vi "get_bias_spectroscopy_sweep_time.vi"() -> (0 "Sweep time (s)":sgl)   [LabVIEW 2021]
uses:
  <userlib>/Nanonis Prog Interface V5/Nanonis Prog Interface.lvlib
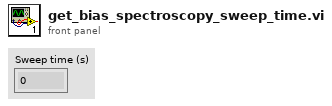
[diagram p1: front panel]
types:
  T1 = cluster{"Z averaging time (s)":sgl, "Z offset (m)":sgl, "Initial settling time (s)":sgl}
  T2 = cluster{"Max. slew rate (V/s)":sgl, "Settling time (s)":sgl, "Integration time (s)":sgl}
  T3 = cluster{"End settling time (s)":sgl, "Z control time (s)":sgl}
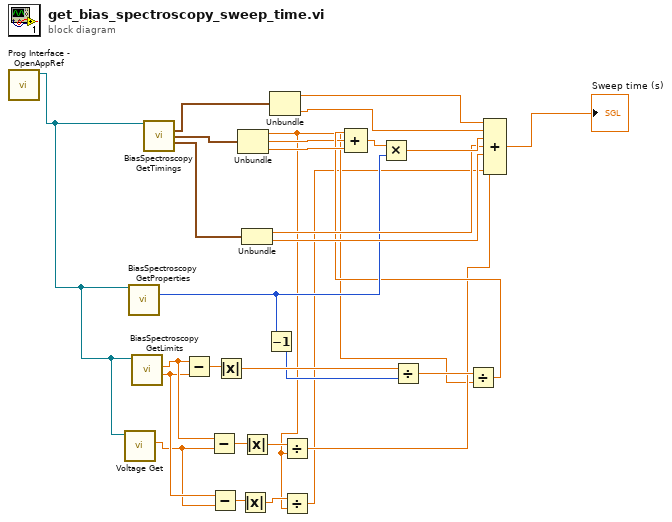
[diagram p0: block diagram]
diagram:
  n1 = call <userlib>:"Prog Interface - OpenAppRef.vi"() -> ("Application reference"=w12:refnum<vi>)  [unwired: 6 in, 1 out]
  n2 = call <userlib>:"Voltage Get.vi"("Application ref in"=w12) -> ("Bias (V)"=w5:sgl)  [unwired: 8 in, 2 out]
  n3 = call <userlib>:"BiasSpectroscopy GetProperties.vi"("Application ref in"=w12) -> ("Number of points"=w17:i32)  [unwired: 7 in, 7 out]
  n4 = call <userlib>:"BiasSpectroscopy GetLimits.vi"("Application ref in"=w12) -> ("End value (V)"=w6:sgl, "Start value (V)"=w11:sgl)  [unwired: 5 in, 2 out]
  n5 = call <userlib>:"BiasSpectroscopy GetTimings.vi"("Application ref in"=w12) -> ("Initialization"=w29:T1, "Sweep Timing"=w28:T2, "End of Sweep"=w27:T3)  [unwired: 10 in, 2 out]
  n6 = Subtract(x=w11, y=w6) -> (x-y=w19:sgl)
  n7 = Subtract(x=w11, y=w5) -> (x-y=w10:sgl)
  n8 = Subtract(x=w6, y=w5) -> (x-y=w4:sgl)
  n9 = Absolute Value(x=w19) -> (abs(x)=w18:sgl)
  n10 = Unbundle(w28) -> ("Max. slew rate (V/s)"=w2:sgl, "Settling time (s)"=w8:sgl, "Integration time (s)"=w26:sgl)
  n11 = Absolute Value(x=w4) -> (abs(x)=w3:sgl)
  n12 = Unbundle(w27) -> ("End settling time (s)"=w22:sgl, "Z control time (s)"=w21:sgl)
  n13 = Absolute Value(x=w10) -> (abs(x)=w9:sgl)
  n14 = Decrement(x=w17) -> (x-1=w13:i32)
  n15 = Unbundle(w29) -> ("Z averaging time (s)"=w16:sgl, "Initial settling time (s)"=w23:sgl)  [unwired: 1 out]
  n16 = Divide(x=w9, y=w2) -> (x/y=w7:sgl)
  n17 = Divide(x=w3, y=w2) -> (x/y=w1:sgl)
  n18 = Divide(x=w18, y=w13) -> (x/y=w15:sgl)
  n19 = Divide(x=w15, y=w2) -> (x/y=w14:sgl)
  n20 = Compound Arithmetic op=ADD(w14, w8, w26) -> (w25:sgl)
  n21 = Multiply(x=w25, y=w17) -> (x*y=w24:sgl)
  n22 = Compound Arithmetic op=ADD(w16, w23, w24, w22, w21, w7, w1) -> (→"Sweep time (s)":sgl)
